vi "Practice with Matlab.vi"() -> ()   [LabVIEW 2015]
uses:
  <vilib>/imath/engines/lvmath/Plug In/_Char/NIMS_CH_character datatype.ctl
  <vilib>/imath/engines/lvmath2/RunTimeEngine/Managers/WorkSpace/UID Generator.vi
  <vilib>/imath/engines/lvmath/Plug In/_Char/NIMS_CH_Character RV to String.vi
  <vilib>/imath/engines/lvmath2/RunTimeEngine/BuiltInFunctions/dir/NIMS_dir.vi
  <vilib>/imath/engines/lvmath/Plug In/_Char/NIMS_CH_String CV to Character 2D.vi
  <instcachedir>/0/NIMS_CH_String CV to Character 2D_4CD47D6F630C6D4AA1E956E0A670B63C.lvgen/NIMS_CH_String CV to Character 2D_4CD47D6F630C6D4AA1E956E0A670B63C_000.vi
  <vilib>/imathl/engines/lvmath/Functions/Error Handling/Create Error.vi
  <vilib>/imath/engines/lvmath2/RunTimeEngine/RangeToken/NIMS_Range_R2 - Integer.vi
  <instcachedir>/0/NIMS_Range_R2 - Integer_E0E86AD0AC6DDF48AE07F756617F7295.lvgen/NIMS_Range_R2 - Integer_E0E86AD0AC6DDF48AE07F756617F7295_000.vi
  <vilib>/imath/engines/lvmath2/RunTimeEngine/CommandStatement/MC_CommandStatement_break.vi
  <vilib>/imath/engines/lvmath2/RunTimeEngine/BuiltInFunctions/fopen/NIMS_fopen(Str).vi
  <vilib>/imath/engines/lvmath/Plug In/_Char/NIMS_CH_Character 1D to U8 1D.vi
  <vilib>/imath/engines/lvmath2/RunTimeSupport/NIMS_Get Scalar_w Error.vi
  <instcachedir>/0/NIMS_Get Scalar_w Error_030D3630995B9340BAE512B6E207FE46.lvgen/NIMS_Get Scalar_w Error_030D3630995B9340BAE512B6E207FE46_010.vi
  <vilib>/imath/engines/lvmath2/RunTimeEngine/BuiltInFunctions/fread/NIMS_fread(I32S,RV,Str,I32S).vi
  <vilib>/imath/engines/lvmath2/RunTimeEngine/RunTimeType/NIMS_RunTimeType_Get Case Value.vi
  <vilib>/imath/engines/lvmath2/RunTimeEngine/RunTimeType/NIMS_RunTimeType_To Numeric.vi
  <instcachedir>/0/NIMS_RunTimeType_To Numeric_A6EDEEF9BCA6644DA2200E5704E38EBF.lvgen/NIMS_RunTimeType_To Numeric_A6EDEEF9BCA6644DA2200E5704E38EBF_003.vi
  <vilib>/imath/engines/lvmath/Plug In/_Char/RunTimeType/NIMS_CH_RunTimeType_To Character 2D.vi
  <vilib>/imath/engines/lvmath2/RunTimeEngine/IndexRead/NIMS M(R2).vi
  <instcachedir>/0/NIMS M(R2)_287818D58BD74005B29FE73CE7602B1A.lvgen/NIMS M(R2)_287818D58BD74005B29FE73CE7602B1A_000.vi
  <vilib>/imath/engines/lvmath2/RunTimeEngine/RunTimeType/NIMS_RunTimeType_From StrictType (excl LVString).vi
  <instcachedir>/0/NIMS_RunTimeType_From StrictType (excl LVString)_CDE8BCA3381BB54ABB7E31EEFBC685C9.lvgen/NIMS_RunTimeType_From StrictType (excl LVString)_CDE8BCA3381BB54ABB7E31EEFBC685C9_009.vi
  <instcachedir>/0/NIMS M(R2)_287818D58BD74005B29FE73CE7602B1A.lvgen/NIMS M(R2)_287818D58BD74005B29FE73CE7602B1A_001.vi
  <instcachedir>/0/NIMS_RunTimeType_From StrictType (excl LVString)_CDE8BCA3381BB54ABB7E31EEFBC685C9.lvgen/NIMS_RunTimeType_From StrictType (excl LVString)_CDE8BCA3381BB54ABB7E31EEFBC685C9_001.vi
  <vilib>/imath/engines/lvmath2/RunTimeEngine/BuiltInFunctions/length/NIMS_length(GM).vi
  <instcachedir>/0/NIMS_length(GM)_47CEC356FCE0482D9BA47DC61C99F2C7.lvgen/NIMS_length(GM)_47CEC356FCE0482D9BA47DC61C99F2C7_000.vi
  <instcachedir>/0/NIMS_length(GM)_47CEC356FCE0482D9BA47DC61C99F2C7.lvgen/NIMS_length(GM)_47CEC356FCE0482D9BA47DC61C99F2C7_004.vi
  <vilib>/imath/engines/lvmath2/RunTimeEngine/RangeToken/NIMS_Range.vi
  <instcachedir>/0/NIMS_Range_5A207EBC289CDB428E903F8A2135C256.lvgen/NIMS_Range_5A207EBC289CDB428E903F8A2135C256_000.vi
  <vilib>/imath/engines/lvmath2/RunTimeSupport/NIMS_Error if Not Equal.vi
  <instcachedir>/0/NIMS_Error if Not Equal_5B27D941BC11DE47BDC877E4E7500DF4.lvgen/NIMS_Error if Not Equal_5B27D941BC11DE47BDC877E4E7500DF4_001.vi
  <vilib>/imath/engines/lvmath2/RunTimeEngine/IndexRead/NIMS M(V,S).vi
  <instcachedir>/0/NIMS M(V,S)_4A7282EC9BD94252BB5D44AC841A97D6.lvgen/NIMS M(V,S)_4A7282EC9BD94252BB5D44AC841A97D6_000.vi
  <instcachedir>/0/NIMS_RunTimeType_From StrictType (excl LVString)_CDE8BCA3381BB54ABB7E31EEFBC685C9.lvgen/NIMS_RunTimeType_From StrictType (excl LVString)_CDE8BCA3381BB54ABB7E31EEFBC685C9_010.vi
  <vilib>/imath/engines/lvmath2/RunTimeEngine/ErrorHandling/NIMS_Create Error From Enums.vi
  <instcachedir>/0/NIMS M(V,S)_4A7282EC9BD94252BB5D44AC841A97D6.lvgen/NIMS M(V,S)_4A7282EC9BD94252BB5D44AC841A97D6_001.vi
  <instcachedir>/0/NIMS_RunTimeType_From StrictType (excl LVString)_CDE8BCA3381BB54ABB7E31EEFBC685C9.lvgen/NIMS_RunTimeType_From StrictType (excl LVString)_CDE8BCA3381BB54ABB7E31EEFBC685C9_006.vi
  <instcachedir>/0/NIMS_RunTimeType_To Numeric_A6EDEEF9BCA6644DA2200E5704E38EBF.lvgen/NIMS_RunTimeType_To Numeric_A6EDEEF9BCA6644DA2200E5704E38EBF_004.vi
  <vilib>/imath/engines/lvmath/Plug In/_Char/RunTimeType/NIMS_CH_RunTimeType_To Character 1D.vi
  <vilib>/imath/engines/lvmath/Functions/Error Handling/MergeErrorsWrapper.vi
  <vilib>/imath/engines/lvmath2/RunTimeEngine/MatrixToken/NIMS_MatrixToken_RV_RV.vi
  <instcachedir>/0/NIMS_MatrixToken_RV_RV_36030E9A8C6DFB4799F99C3FA1CC442B.lvgen/NIMS_MatrixToken_RV_RV_36030E9A8C6DFB4799F99C3FA1CC442B_002.vi
  <vilib>/imath/engines/lvmath/Plug In/_Char/NIMS_CH_U8 1D to Character 1D.vi
  <instcachedir>/0/NIMS_MatrixToken_RV_RV_36030E9A8C6DFB4799F99C3FA1CC442B.lvgen/NIMS_MatrixToken_RV_RV_36030E9A8C6DFB4799F99C3FA1CC442B_003.vi
  Documents/LabVIEW Data/MathScriptVIs/MCStatic_35241984432_5626021b76c646a419d02b10edb48605.vi
  <instcachedir>/0/MCStatic_35241984432_5626021b76c646a419d02b10edb48605_6CA23249ABC7A54B87A14E8691C6872E.lvgen/MCStatic_35241984432_5626021b76c646a419d02b10edb48605_6CA23249ABC7A54B87A14E8691C6872E_000.vi
  <vilib>/imath/engines/lvmath2/RunTimeEngine/BuiltInFunctions/atan2/NIMS_atan2(A,A).vi
  <instcachedir>/0/NIMS_atan2(A,A)_E4477B144D76734483D5B13799B9510C.lvgen/NIMS_atan2(A,A)_E4477B144D76734483D5B13799B9510C_004.vi
  <vilib>/imath/engines/lvmath2/RunTimeEngine/Managers/SymbolTable/Clear UID.vi
  <vilib>/imath/engines/lvmath2/RunTimeEngine/ErrorHandling/NIMS_Finalize Error.vi
  <vilib>/Utility/file.llb/Read From Spreadsheet File (DBL).vi
  <vilib>/imath/engines/lvmath2/RunTimeEngine/LocalVariableDefStatement/MC_LocalVariableDefStatement_Display.vi
  <vilib>/imath/engines/lvmath2/RunTimeEngine/BuiltInFunctions/fopen/NIMS_fopen(Str,Enum).vi
  <vilib>/imath/engines/lvmath2/RunTimeEngine/NodeEndStatement/NIMS_NodeEndStatement_Output.vi
  <instcachedir>/0/NIMS_NodeEndStatement_Output_53EC0D466D134D7ABD903AC30B43404B.lvgen/NIMS_NodeEndStatement_Output_53EC0D466D134D7ABD903AC30B43404B_011.vi
  <instcachedir>/0/NIMS_NodeEndStatement_Output_53EC0D466D134D7ABD903AC30B43404B.lvgen/NIMS_NodeEndStatement_Output_53EC0D466D134D7ABD903AC30B43404B_010.vi
  Documents/LabVIEW Data/MathScriptVIs/MCStatic_35241984432_36dd5741f7b4df6594758ef2aa7f08ac.vi
  <instcachedir>/0/MCStatic_35241984432_36dd5741f7b4df6594758ef2aa7f08ac_942583B371DBC64A92E079298D9E649B.lvgen/MCStatic_35241984432_36dd5741f7b4df6594758ef2aa7f08ac_942583B371DBC64A92E079298D9E649B_000.vi
  <vilib>/imath/engines/lvmath2/RunTimeEngine/UserFunctionToken/NIMS_UserFunction_CondDefined.vi
  <instcachedir>/0/NIMS_UserFunction_CondDefined_94700CD48F9208418FC93D629E647FB6.lvgen/NIMS_UserFunction_CondDefined_94700CD48F9208418FC93D629E647FB6_000.vi
  <instcachedir>/0/NIMS_RunTimeType_From StrictType (excl LVString)_CDE8BCA3381BB54ABB7E31EEFBC685C9.lvgen/NIMS_RunTimeType_From StrictType (excl LVString)_CDE8BCA3381BB54ABB7E31EEFBC685C9_000.vi
  <instcachedir>/0/NIMS_UserFunction_CondDefined_94700CD48F9208418FC93D629E647FB6.lvgen/NIMS_UserFunction_CondDefined_94700CD48F9208418FC93D629E647FB6_001.vi
  <vilib>/imath/engines/lvmath2/RunTimeEngine/VariableToken/NIMS_VariableToken_CondDefined.vi
  <instcachedir>/0/NIMS_VariableToken_CondDefined_9A0647DCF861C347AE2CF513BAEE419F.lvgen/NIMS_VariableToken_CondDefined_9A0647DCF861C347AE2CF513BAEE419F_005.vi
  <instcachedir>/0/NIMS_NodeEndStatement_Output_53EC0D466D134D7ABD903AC30B43404B.lvgen/NIMS_NodeEndStatement_Output_53EC0D466D134D7ABD903AC30B43404B_005.vi
  MATLAB/RUS/CircleFitByPratt.m
  MATLAB/RUS/lorentzfit_general_forLabVIEW.m
  MATLAB/RUS/lfun3c.m
  MATLAB/RUS/lfun3c_dispersive.m
  <vilib>/imath/engines/lvmath2/RunTimeEngine/Managers/SymbolTable/NIMS_WorkSpace.lvlib
panel:
  out "Data and BG":cluster{"all rows":dbl[], "all rows":dbl[]}[](graph)
  out "best fit params":dbl[](array[numeric])
  out "Subset and Fit":T1(graph)
  out "contents 2":string
  out "contents":string[](array[string])
  out "fileID":i32
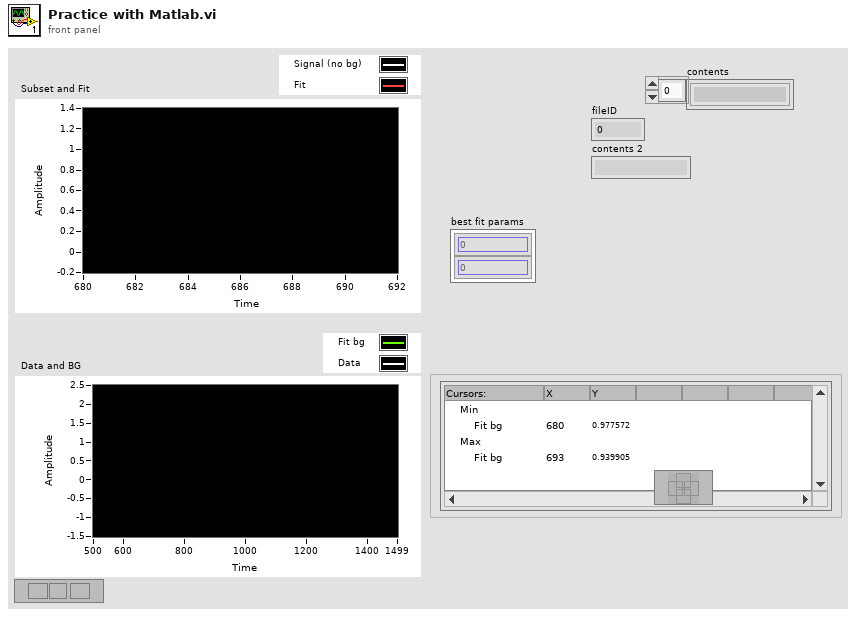
[diagram p1: front panel]
types:
  T1 = cluster{"X subset":dbl[], "best nonlinear fit":dbl[]}[]
  T2 = typedef "NIMS_CH_character datatype.ctl" = cluster{"Numeric":u8}
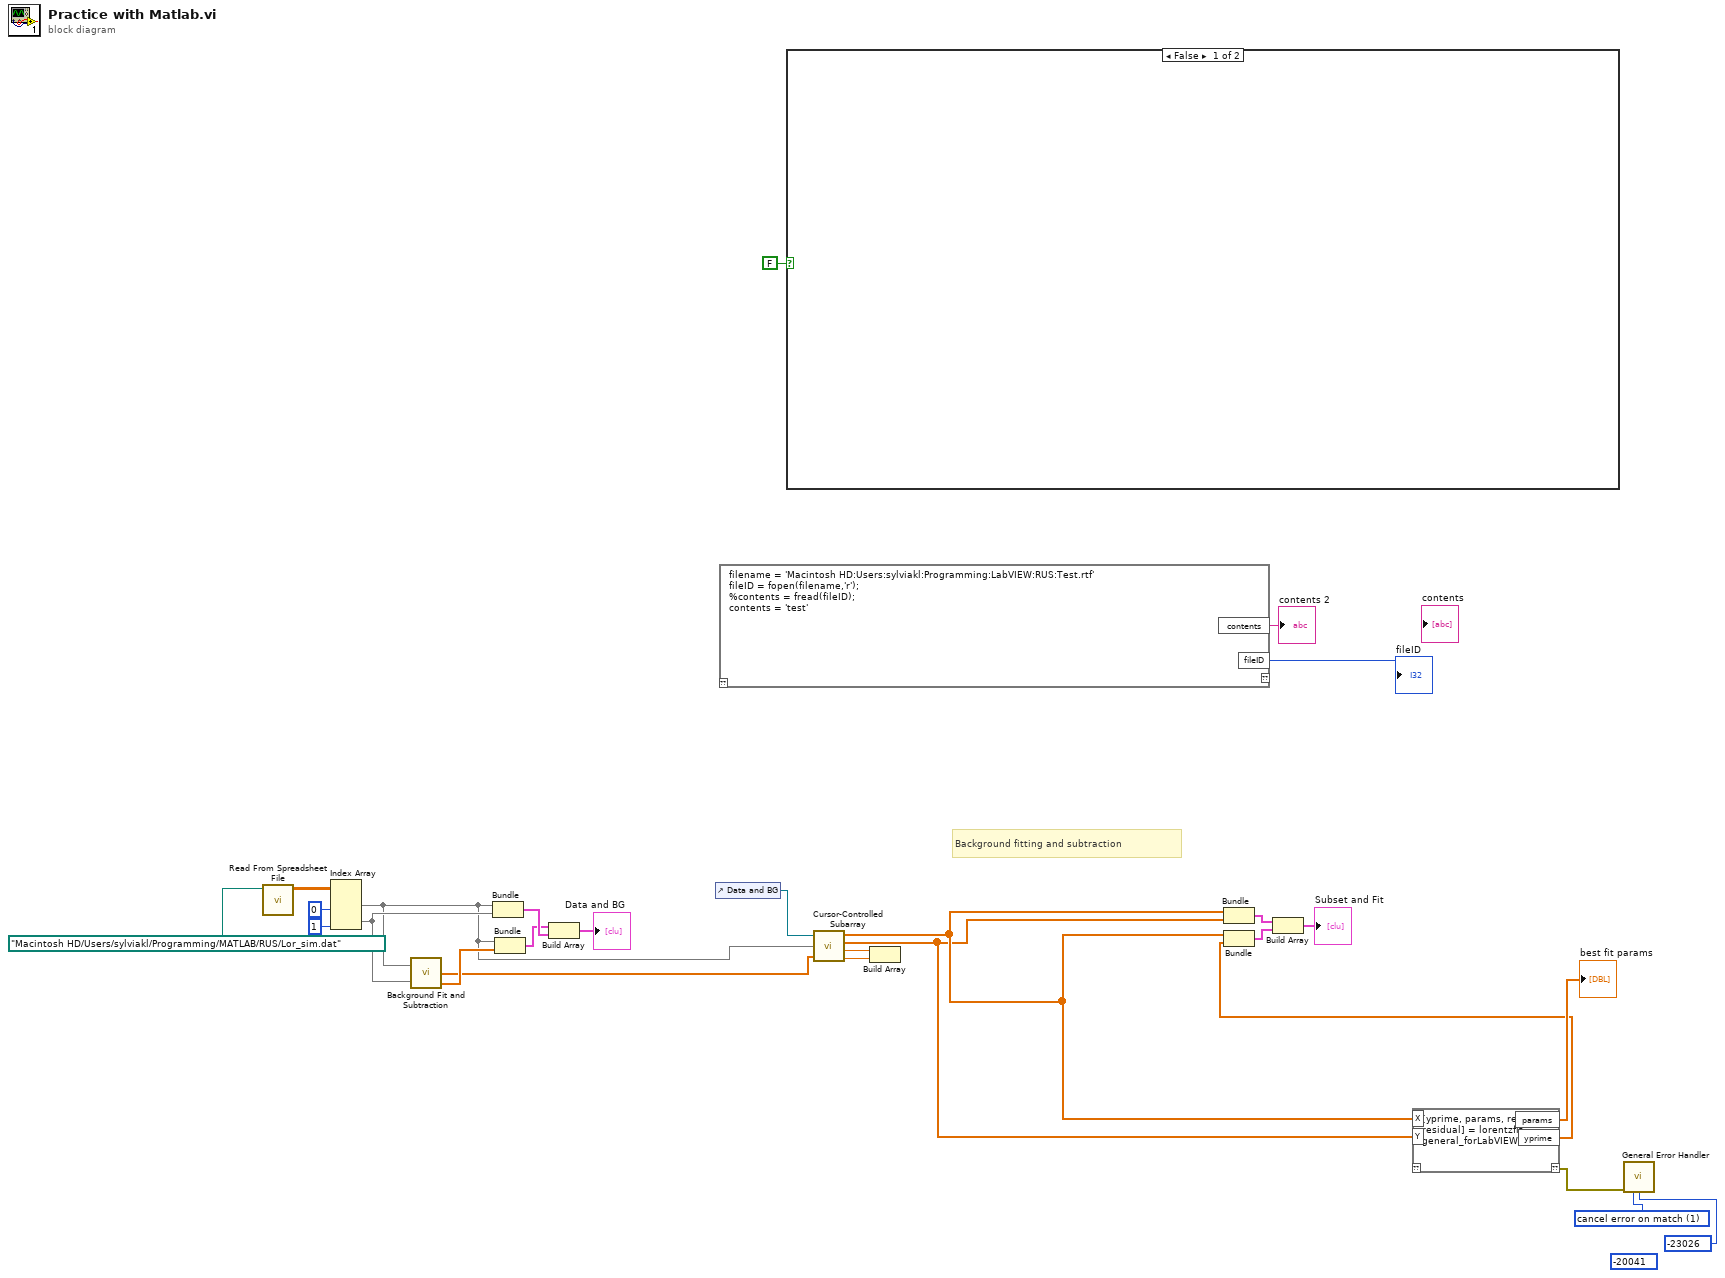
[diagram p0: block diagram]
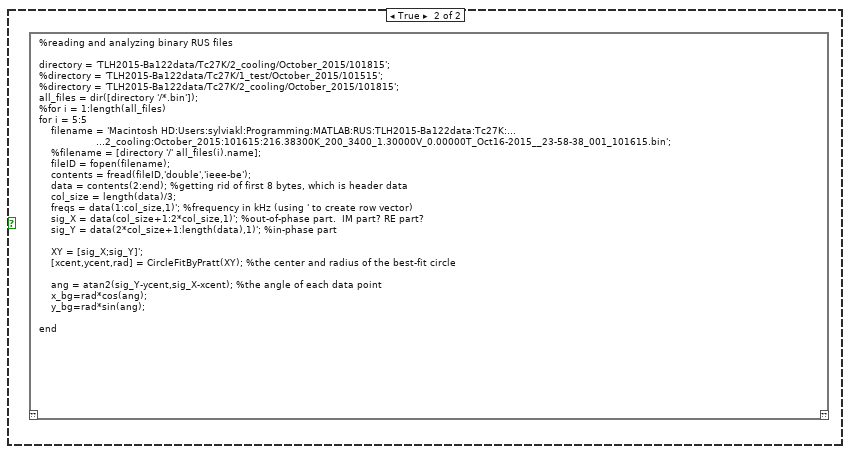
[diagram p2: hidden frame]
diagram:
  (unwired) -20041 ("[exception code]")
  w3 = 1 items=["no exception", "cancel error on match", "set error on match"] ("[exception action] (none:0)")
  # "Background fitting and subtraction"
  n1 = call-poly <vilib>:"Read From Spreadsheet File.vi"("file path (dialog if empty)"=path "/Macintosh HD/Users/sylviakl/Programming/MATLAB/RUS/Lor_sim.dat" ("Path")) -> ("all rows"=w17:dbl[][])  [unwired: 6 in, 4 out]
  n2 = Index Array(array=w17, index (col) #1=0 ("disabled index (col)"), index (col) #2=1 ("index (col)")) -> (element #1=w9:dbl[], element #2=w16:dbl[])  [unwired: 2 in]
  n3 = call "Background Fit and Subtraction.vi"("X"=w9, "Y"=w16) -> ("signal"=w10:dbl[], "background"=w14:dbl[])  [unwired: 1 out]
  n4 = Bundle("all rows"=w9, "all rows"=w16) -> (w13:cluster{"all rows":dbl[], "all rows":dbl[]})  [unwired: 1 in]
  n5 = Bundle("all rows"=w9, "background"=w14) -> (w12:cluster{"all rows":dbl[], "background":dbl[]})  [unwired: 1 in]
  n6 = Build Array(w12, w13) -> (→"Data and BG":cluster{"all rows":dbl[], "all rows":dbl[]}[])
  n7 = control-ref of="Data and BG"() -> (w8:refnum<vi>)
  n8 = mathscript code="filename = 'Macintosh HD:Users:sylviakl:Programming:LabVIEW:RUS:Test.rtf'\nfileID = fopen(filename,'r');\n%contents = fread(fileID);\ncontents = 'test'"() -> ("contents"=→"contents 2":string, "fileID"=→"fileID":i32)  [unwired: 1 in, 1 out]
  n9 = case shown="False" FALSE {
    frame False {
    }
    frame True {
      n10 = mathscript code="%reading and analyzing binary RUS files\n\ndirectory = 'TLH2015-Ba122data/Tc27K/2_cooling/October_2015/101815';\n%directory = 'TLH2015-Ba122data/Tc27K/1_test/October_2015/101515';\n%directory = 'TLH2015-Ba122data/Tc27K/2_cooling/October_2015/101815';\nall_files = dir([directory '/*.bin']);\n%for i = 1:length(all_files)\nfor i = 5:5\n    filename = 'Macintosh HD:Users:sylviakl:Programming:MATLAB:RUS:TLH2015-Ba122data:Tc27K:...\n                   ...2_cooling:October_2015:101615:216.38300K_200_3400_1.30000V_0.00000T_Oct16-2015__23-58-38_001_101615.bin';\n    %filename = [directory '/' all_files(i).name];\n    fileID = fopen(filename);\n    contents = fread(fileID,'double','ieee-be');\n    data = contents(2:end); %getting rid of first 8 bytes, which is header data\n    col_size = length(data)/3;\n    freqs = data(1:col_size,1)'; %frequency in kHz (using ' to create row vector)\n    sig_X = data(col_size+1:2*col_size,1)'; %out-of-phase part.  IM part? RE part?\n    sig_Y = data(2*col_size+1:length(data),1)'; %in-phase part\n\n    XY = [sig_X;sig_Y]';\n    [xcent,ycent,rad] = CircleFitByPratt(XY); %the center and radius of the best-fit circle\n\n    ang = atan2(sig_Y-ycent,sig_X-xcent); %the angle of each data point\n    x_bg=rad*cos(ang);\n    y_bg=rad*sin(ang);\n\nend"() -> ()  [unwired: 1 in, 1 out]
    }
  }
  n11 = call "Cursor-Controlled Subarray.vi"("cursor graph"=w8, "X"=w9, "Y"=w10) -> ("X subset"=w7:dbl[], "Y subset"=w6:dbl[], "cursor avg"=w20:dbl, "cursor diff"=w21:dbl)
  n12 = Build Array(w20, w21) -> ()  [unwired: 1 out]
  n13 = Bundle("X subset"=w7, "Y subset"=w6) -> (w23:cluster{"X subset":dbl[], " Y subset":dbl[]})  [unwired: 1 in]
  n14 = mathscript code="[yprime, params, resnorm, residual] = lorentzfit_general_forLabVIEW(X,Y)"("X"=w7, "Y"=w6) -> ("??"=w2:errorcluster, "params"=→"best fit params":dbl[], "yprime"=w4:dbl[])  [unwired: 1 in]
  n15 = Bundle("X subset"=w7, "yprime"=w4) -> (w22:cluster{"X subset":dbl[], "yprime":dbl[]})  [unwired: 1 in]
  n16 = Build Array(w23, w22) -> (→"Subset and Fit":cluster{"X subset":dbl[], "yprime":dbl[]}[])
  n17 = call <vilib>:"General Error Handler.vi"("error in (no error)"=w2, "[exception action] (none:0)"=w3, "[exception code]"=-23026) -> ()  [unwired: 8 in, 5 out]
